vi "Final_result.vi"(11 "Boolean array":bool[](array[boolean])) -> (1 "logical AND":bool, 2 "Status Color":u32, 3 "Status":string)   [LabVIEW 2021]
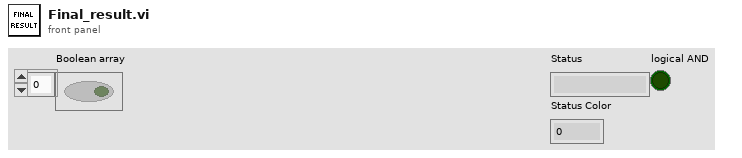
[diagram p1: front panel]
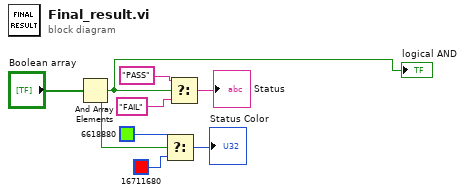
[diagram p0: block diagram]
diagram:
  n1 = And Array Elements(Boolean array="Boolean array") -> (logical AND=w4:bool)
  "logical AND" <- w4
  n2 = Select(t=u32 6618880 ("Text.Text Colors:BG Color"), s=w4, f=u32 16711680 ("Text.Text Colors:BG Color")) -> (s? t:f=→"Status Color":u32)
  n3 = Select(t="PASS", s=w4, f="FAIL") -> (s? t:f=→"Status":string)
